vi "Pixel1.1.vi"() -> ()   [LabVIEW 2018]
panel:
  in  "Start Game/Robots turn":bool
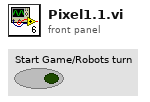
[diagram p1: front panel]
types:
  T1 = enum16{"Child's Turn", "Robot's Turn", "Waiting State", "Game Over"}
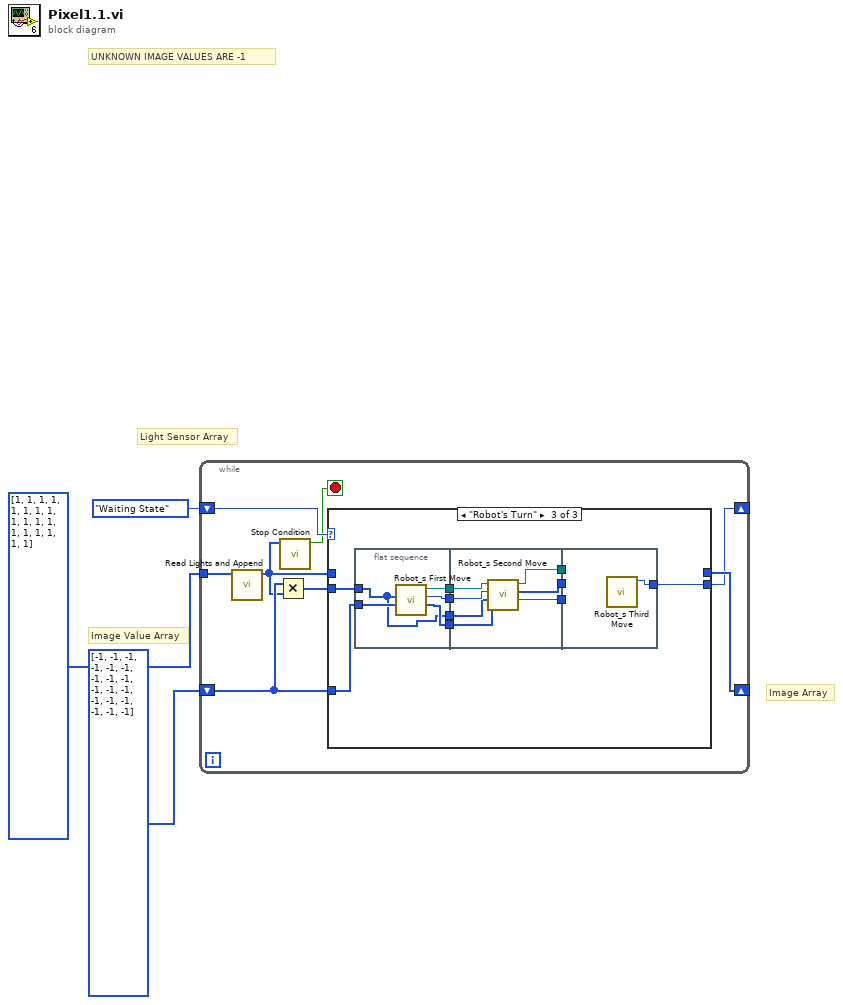
[diagram p0: block diagram]
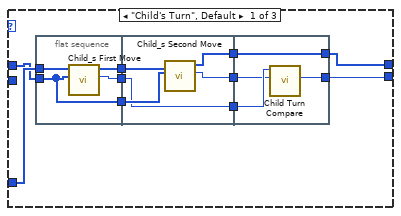
[diagram p2: hidden frame]
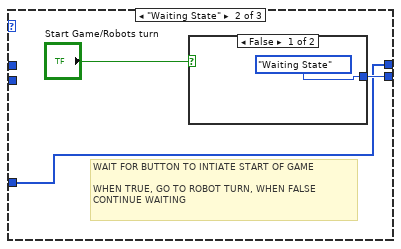
[diagram p3: hidden frame]
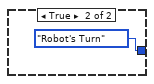
[diagram p4: hidden frame]
diagram:
  # "Image Array"
  # "UNKNOWN IMAGE VALUES ARE -1"
  # "Light Sensor Array"
  # "Image Value Array"
  n1 = while {
    shift-right: [w7] -> _
    shift-left: T1."Waiting State" -> [w11]
    shift-right: [w8] -> _
    shift-left: i32[] [-1, -1, -1, -1, -1, -1, -1, -1, -1, -1, -1, -1, -1, -1, -1, -1, -1, -1] ("Array") -> [w5]
    tunnel: i32[] [1, 1, 1, 1, 1, 1, 1, 1, 1, 1, 1, 1, 1, 1, 1, 1, 1, 1] ("Array") -> [w6]
    stop <- w10 stop-if-true
    n2 = call "Read Lights and Append.vi"("Input Array"=w6) -> ("Output Array"=w4:i32[])  [unwired: 7 in]
    n3 = Multiply(x=w5, y=w4) -> (x*y=w9:i32[])
    n4 = call "Stop Condition.vi"("Light Sensor Array"=w4) -> ("element"=w10:bool)  [unwired: 10 in]
    n5 = case shown="\"Robot's Turn\"" w11 {
      tunnel: w9 -> [_ _ w49]
      tunnel: [w16 w35 _] -> w8
      tunnel: [w12 w36 w46] -> w7
      tunnel: w5 -> [w21 w35 w45]
      tunnel: w4 -> [w20 _ _]
      frame "Child's Turn", Default {
        n6 = flat-sequence {
          tunnel: w21 -> [w25]
          tunnel: w20 -> [w23]
          tunnel: [w24] -> w19
          tunnel: [w23] -> w18
          tunnel: [w22] -> w15
          tunnel: w19 -> [w30]
          tunnel: w18 -> [w29]
          tunnel: [w28] -> w17
          tunnel: w15 -> [w27]
          tunnel: [w27] -> w14
          tunnel: [w26] -> w13
          tunnel: [w34] -> w16
          tunnel: w17 -> [w34]
          tunnel: w14 -> [w33]
          tunnel: w13 -> [w32]
          tunnel: [w31] -> w12
          frame #0 {
            n7 = call "Child_s First Move.vi"("Old Light Sensor Array"=w23, "Current Image Array"=w25) -> ("Image Value From First Turn"=w22:i32, "Output Image Array"=w24:i32[])  [unwired: 8 in]
          }
          frame #1 {
            n8 = call "Child_s Second Move.vi"("Old Light Sensor Array"=w29, "Current Image Array"=w30) -> ("Image Value From Second Turn"=w26:i32, "Output Image Array"=w28:i32[])  [unwired: 8 in]
          }
          frame #2 {
            n9 = call "Child Turn Compare.vi"("Image Value from Second Move"=w32, "Image value from First Move"=w33) -> ("Next Move"=w31:T1)  [unwired: 9 in]
          }
        }
      }
      frame "Waiting State" {
        # "WAIT FOR BUTTON TO INTIATE START OF GAME\n\nWHEN TRUE, GO TO ROBOT TURN, WHEN FALSE \nCONTINUE WAITING"
        n10 = case shown="False" "Start Game/Robots turn" {
          tunnel: [T1."Waiting State" T1."Robot's Turn"] -> w36
          frame False {
          }
          frame True {
          }
        }
      }
      frame "Robot's Turn" {
        n11 = flat-sequence {
          tunnel: w49 -> [w50]
          tunnel: [w54] -> w48
          tunnel: [w53] -> w47
          tunnel: w45 -> [w52]
          tunnel: [w51] -> w44
          tunnel: [w50] -> w43
          tunnel: w48 -> [w61]
          tunnel: w47 -> [w58]
          tunnel: w44 -> [w60]
          tunnel: w43 -> [w59]
          tunnel: [w57] -> w42
          tunnel: [w56] -> w41
          tunnel: [w55] -> w40
          tunnel: [w62] -> w46
          tunnel: w42 -> [_]
          tunnel: w41 -> [_]
          tunnel: w40 -> [_]
          frame #0 {
            n12 = call "Robot_s First Move.vi"("Current Image Array 2"=w52, "In Play Array"=w50) -> ("Output Image Array"=w53:i32[], "Index From First Move"=w51:i32, "VISA Refnum out"=w54:refnum<visa-resource-name>)  [unwired: 6 in, 1 out]
          }
          frame #1 {
            n13 = call "Robot_s Second Move.vi"("Current Image Array"=w58, "In Play Array"=w59, "Index from First Move"=w60, "VISA Refnum in"=w61) -> ("Image Value from Second Turn"=w55:i32, "Output Image Array"=w56:i32[], "VISA Refnum out"=w57:refnum<visa-resource-name>)  [unwired: 4 in]
          }
          frame #2 {
            n14 = call "Robot_s Third Move.vi"() -> ("Next Move"=w62:enum16{"Child's Turn", "Robot's Turn"})  [unwired: 11 in]
          }
        }
      }
    }
  }
